vi "call test.vi"() -> ()   [LabVIEW 2022 SP3]
uses:
  gitlab/nanotecsteppercontroller/NanotecStepperController/x64/Debug/Nanotec Controller States Enum.ctl
  NanoLibDLL/build/x64/Release/NanoLibDLL.dll
panel:
  out "error in (no error)":errorcluster
  in  "Scan Port":bool
  in  "Devices":i32(listbox)
  out "Busy":bool
  out "error out inner":errorcluster
  out "status":i32
  in  "Connect Device":bool
  in  "Ports":i32(listbox)
  out "Controller ptr":u64
  in  "Stop":bool
  in  "Close Controller":bool
  in  "Open Port":bool
  in  "Get Ports":bool
  in  "AutoSetupMotPams":bool
  out "error out":errorcluster
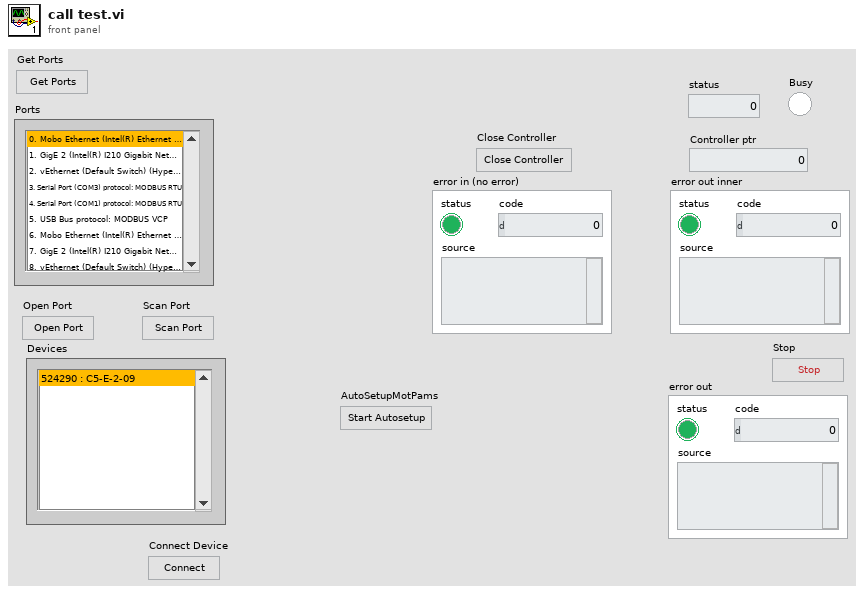
[diagram p1: front panel]
types:
  T1 = typedef "Nanotec Controller States Enum.ctl" = enum16{"Connect Device", "Wait", "Close Controller", "ScanBus", "OpenPort", "GetPorts", "AutoSetupMotPams"}
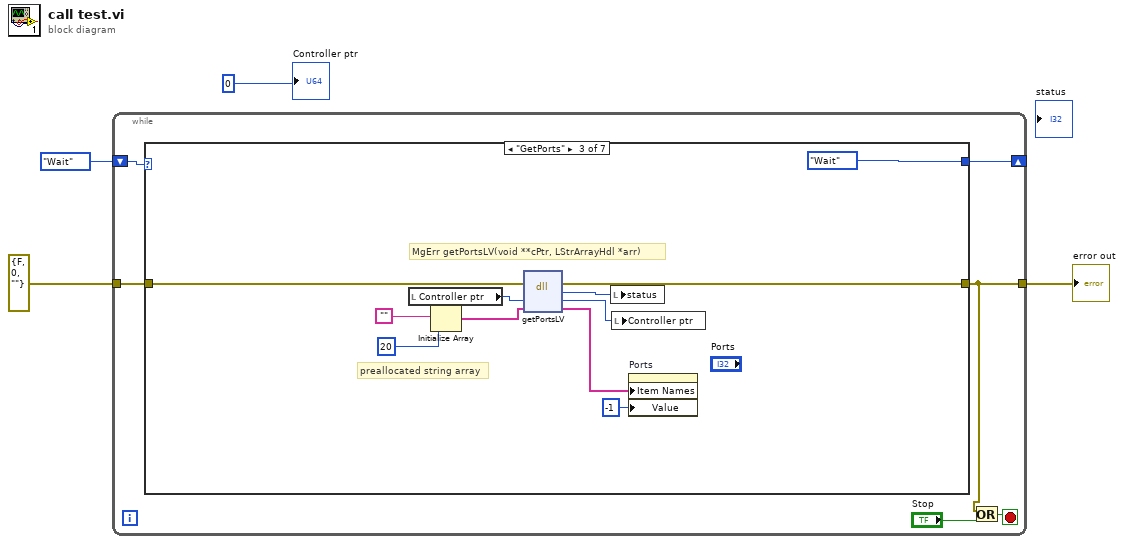
[diagram p0: block diagram]
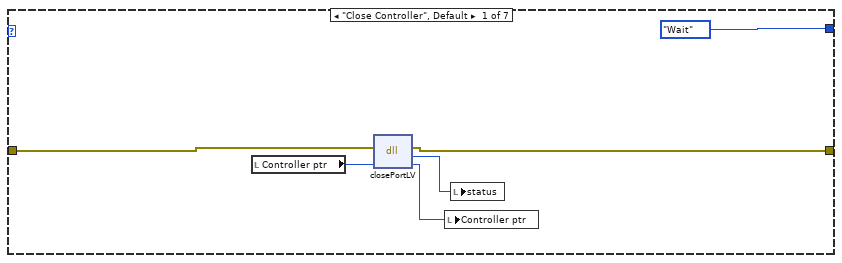
[diagram p2: hidden frame]
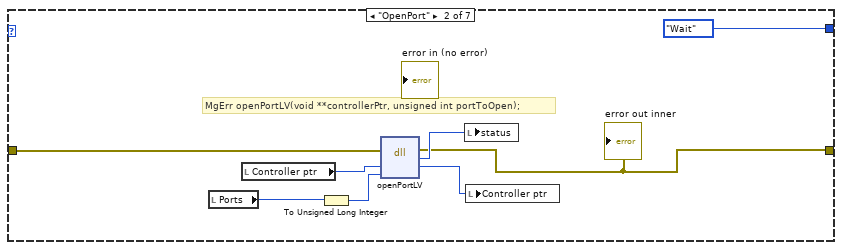
[diagram p3: hidden frame]
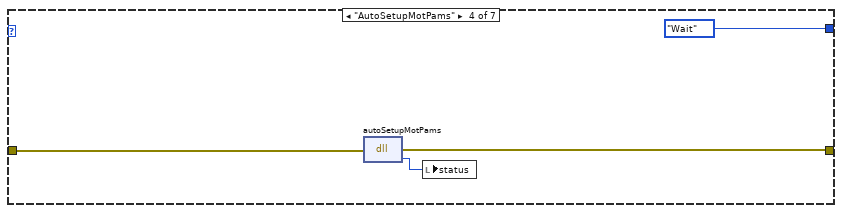
[diagram p4: hidden frame]
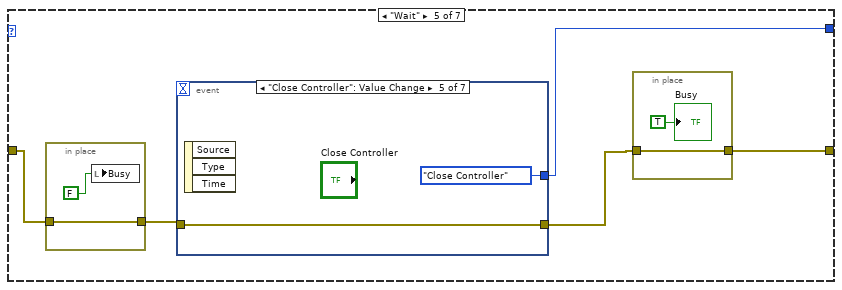
[diagram p5: hidden frame]
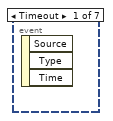
[diagram p6: hidden frame]
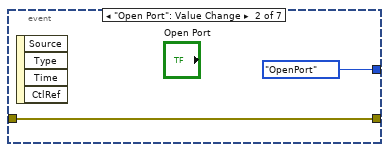
[diagram p7: hidden frame]
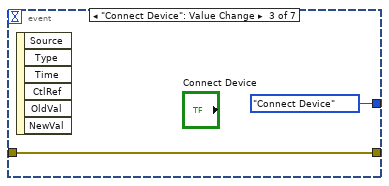
[diagram p8: hidden frame]
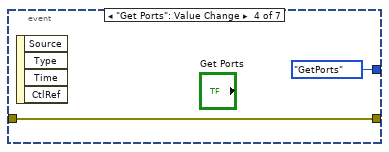
[diagram p9: hidden frame]
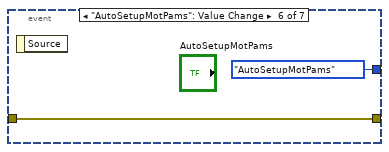
[diagram p10: hidden frame]
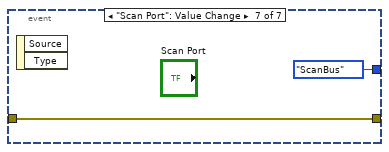
[diagram p11: hidden frame]
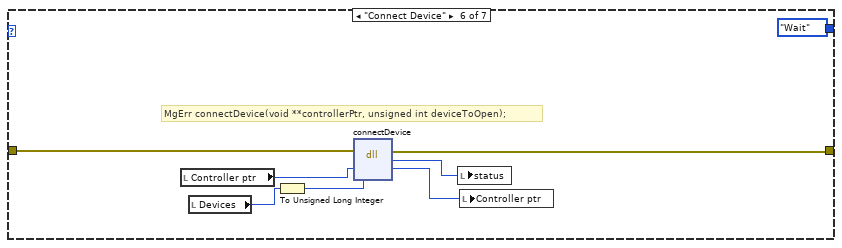
[diagram p12: hidden frame]
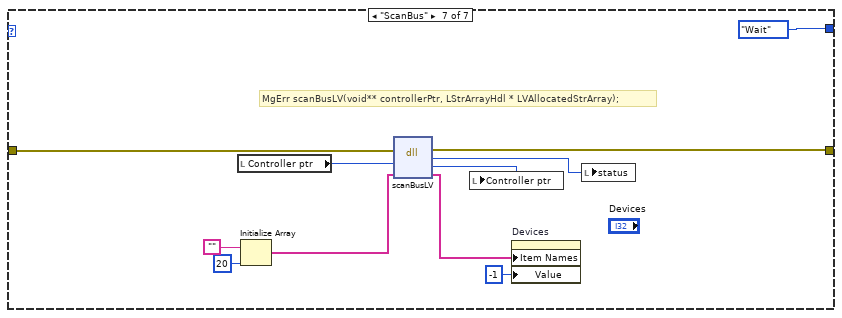
[diagram p13: hidden frame]
diagram:
  n1 = while {
    tunnel: [w6] -> w4
    tunnel: errorcluster {"status"=FALSE, "code"=0, "source"=""} ("error in (no error)") -> [w9]
    shift-right: [w8] -> _
    shift-left: Nanotec_Controller_States_Enum."Wait" -> [w10]
    stop <- w7 stop-if-true
    n2 = case shown="\"GetPorts\"" w10 {
      tunnel: [w14 w18 w30 w37 w42 w65 w75] -> w6
      tunnel: w9 -> [w15 w22 w31 w38 w41 w66 w76]
      tunnel: [Nanotec_Controller_States_Enum."Wait" Nanotec_Controller_States_Enum."Wait" Nanotec_Controller_States_Enum."Wait" Nanotec_Controller_States_Enum."Wait" w44 Nanotec_Controller_States_Enum."Wait" Nanotec_Controller_States_Enum."Wait"] -> w8
      frame "Close Controller", Default {
        n3 = local read "Controller ptr"() -> (w11:u64)
        n4 = dll-call lib="D:/git/NanoLib-Labview-Wrapper/NanoLibDLL/build/x64/Release/NanoLibDLL.dll" fn="closePortLV"(error in=w15, "objPtr"=w11) -> (error out=w14:errorcluster, "return type"=w13:i32, "objPtr"=w12:u64)  [unwired: 2 in, 1 out]
        n5 = local write "Controller ptr"(w12) -> ()
        n6 = local write "status"(w13) -> ()
      }
      frame "OpenPort" {
        # "MgErr openPortLV(void **controllerPtr, unsigned int portToOpen);"
        n7 = local read "Ports"() -> (w23:i32)
        n8 = local read "Controller ptr"() -> (w20:u64)
        n9 = To Unsigned Long Integer(number=w23) -> (unsigned 32bit integer=w21:u32)
        n10 = dll-call lib="D:/git/NanoLib-Labview-Wrapper/NanoLibDLL/build/x64/Release/NanoLibDLL.dll" fn="openPortLV"(error in=w22, "objPtr"=w20, "portToOpen"=w21) -> (error out=w18:errorcluster, "return type"=w19:i32, "objPtr"=w17:u64)  [unwired: 3 in, 1 out]
        "error out inner" <- w18
        n11 = local write "status"(w19) -> ()
        n12 = local write "Controller ptr"(w17) -> ()
      }
      frame "GetPorts" {
        # "MgErr getPortsLV(void **cPtr, LStrArrayHdl *arr)"
        # "preallocated string array"
        n13 = local read "Controller ptr"() -> (w26:u64)
        n14 = Initialize Array("", 20 ("dimension size")) -> (w28:string[])
        n15 = dll-call lib="D:/git/NanoLib-Labview-Wrapper/NanoLibDLL/build/x64/Release/NanoLibDLL.dll" fn="getPortsLV"(error in=w31, "objPtr"=w26, "strArray"=w28) -> (error out=w30:errorcluster, "return type"=w29:i32, "objPtr"=w25:u64, "strArray"=w27:string[])  [unwired: 2 in, 1 out]
        n16 = local write "status"(w29) -> ()
        n17 = local write "Controller ptr"(w25) -> ()
        n18 = property on="Ports" class="LstBox (strict)"("Item Names"=w27, "Value"=-1 ("Interfaces")) -> ()  [unwired: 2 in, 2 out]
      }
      frame "AutoSetupMotPams" {
        n19 = dll-call lib="D:/git/NanoLib-Labview-Wrapper/NanoLibDLL/build/x64/Release/NanoLibDLL.dll" fn="autoSetupMotPams"(error in=w38) -> (error out=w37:errorcluster, "return type"=w36:i32)  [unwired: 2 in, 1 out]
        n20 = local write "status"(w36) -> ()
      }
      frame "Wait" {
        n21 = in-place {
          in-place-border: w41 -> [w45]
          in-place-border: [w45] -> w40
          n22 = local write "Busy"(FALSE ("Busy")) -> ()
        }
        n23 = event shown="[4] \"Close Controller\": Value Change" {
          selector: _ -> [_ _ _ _ _ _ _]
          dyn-events: _ -> [_ _ _ _ _ _ _]
          timeout: _ -> [_ _ _ _ _ _ _]
          tunnel: [_ Nanotec_Controller_States_Enum."OpenPort" Nanotec_Controller_States_Enum."Connect Device" Nanotec_Controller_States_Enum."GetPorts" Nanotec_Controller_States_Enum."Close Controller" Nanotec_Controller_States_Enum."AutoSetupMotPams" Nanotec_Controller_States_Enum."ScanBus"] -> w44
          tunnel: w40 -> [_ w49 w52 w53 w55 w57 w60]
          tunnel: [_ w49 w52 w53 w55 w57 w60] -> w43
          event Timeout {
            n24 = event-data() -> ()  [unwired: 1 in, 3 out]
          }
          event "Open Port": Value Change {
            n25 = event-data() -> ()  [unwired: 1 in, 4 out]
          }
          event "Connect Device": Value Change {
            n26 = event-data() -> ()  [unwired: 1 in, 6 out]
          }
          event "Get Ports": Value Change {
            n27 = event-data() -> ()  [unwired: 1 in, 4 out]
          }
          event "Close Controller": Value Change {
            n28 = event-data() -> ()  [unwired: 1 in, 3 out]
          }
          event "AutoSetupMotPams": Value Change {
            n29 = event-data() -> ()  [unwired: 1 in, 1 out]
          }
          event "Scan Port": Value Change {
            n30 = event-data() -> ()  [unwired: 1 in, 2 out]
          }
        }
        n31 = in-place {
          in-place-border: w43 -> [w48]
          in-place-border: [w48] -> w42
          "Busy" <- TRUE ("Busy")
        }
      }
      frame "Connect Device" {
        # "MgErr connectDevice(void **controllerPtr, unsigned int deviceToOpen);"
        n32 = local read "Controller ptr"() -> (w64:u64)
        n33 = local read "Devices"() -> (w67:i32)
        n34 = To Unsigned Long Integer(number=w67) -> (unsigned 32bit integer=w61:u32)
        n35 = dll-call lib="D:/git/NanoLib-Labview-Wrapper/NanoLibDLL/build/x64/Release/NanoLibDLL.dll" fn="connectDevice"(error in=w66, "objPtr"=w64, "deviceToOpen"=w61) -> (error out=w65:errorcluster, "return type"=w63:i32, "objPtr"=w62:u64)  [unwired: 3 in, 1 out]
        n36 = local write "status"(w63) -> ()
        n37 = local write "Controller ptr"(w62) -> ()
      }
      frame "ScanBus" {
        # "MgErr scanBusLV(void** controllerPtr, LStrArrayHdl * LVAllocatedStrArray);"
        n38 = local read "Controller ptr"() -> (w72:u64)
        n39 = Initialize Array("", 20 ("dimension size")) -> (w74:string[])
        n40 = dll-call lib="D:/git/NanoLib-Labview-Wrapper/NanoLibDLL/build/x64/Release/NanoLibDLL.dll" fn="scanBusLV"(error in=w76, "objPtr"=w72, "devStrArray"=w74) -> (error out=w75:errorcluster, "return type"=w70:i32, "objPtr"=w71:u64, "devStrArray"=w73:string[])  [unwired: 2 in, 1 out]
        n41 = local write "Controller ptr"(w71) -> ()
        n42 = property on="Devices" class="LstBox (strict)"("Item Names"=w73, "Value"=-1 ("Interfaces")) -> ()  [unwired: 2 in, 2 out]
        n43 = local write "status"(w70) -> ()
      }
    }
    n44 = Or(x=w6, y="Stop") -> (x .or. y?=w7:bool)
  }
  "error out" <- w4
  "Controller ptr" <- u64 0
